vi "find device.vi"(8 "error in (no error)":errorcluster, 11 "USB-6000 in":refnum<class "USB-6000.lvclass">) -> (0 "error out":errorcluster, 3 "USB-6000 out":refnum<class "USB-6000.lvclass">)   [LabVIEW 2025, in "USB IO.lvlib" / "USB-6000.lvclass"]
uses:
  USB-6000.lvclass
  USB-6000.lvclass/USB-6000.ctl
  USB IO.lvclass
  <resource>/objmgr/daqmx.rc
panel:
  out "DO.Lines":tag[](array[tag])
  out "AI.PhysicalChans":tag[](array[tag])
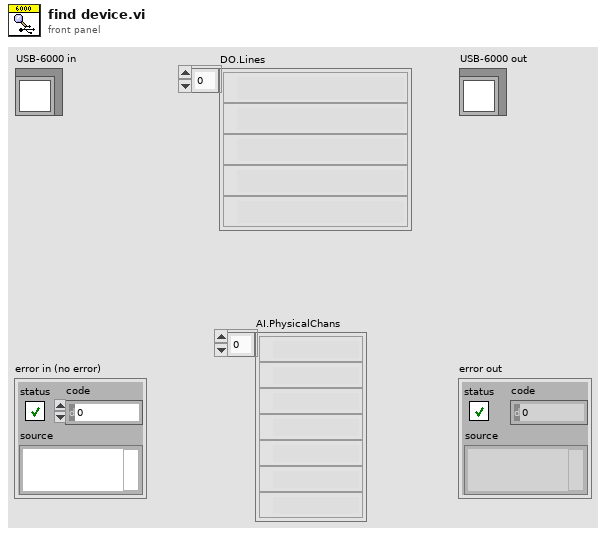
[diagram p1: front panel]
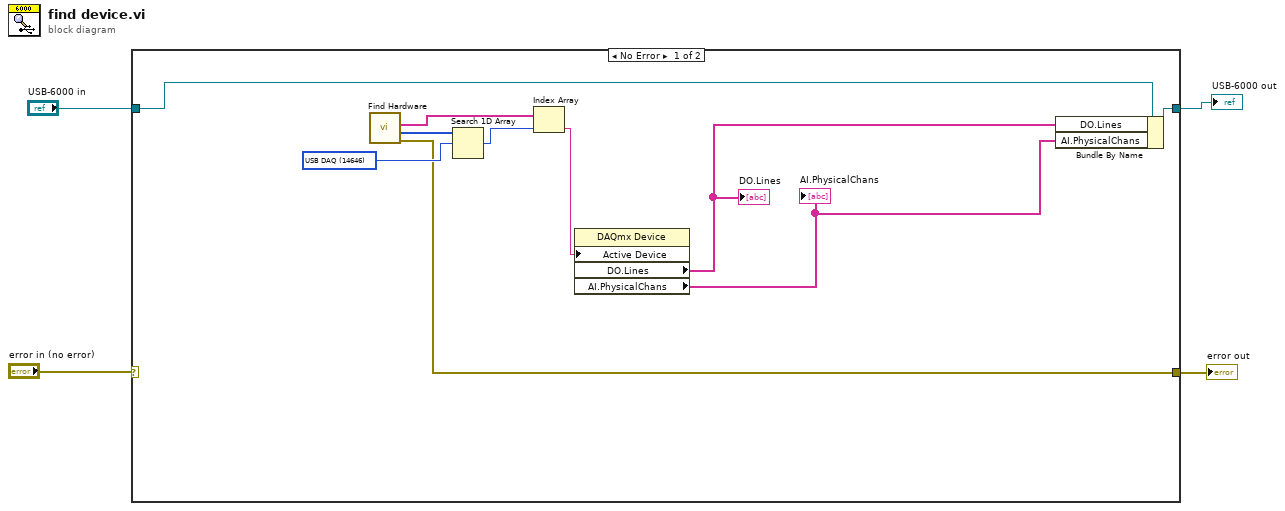
[diagram p0: block diagram]
diagram:
  n1 = case shown="No Error" "error in (no error)" {
    selector: "error in (no error)" -> [_ w16]
    tunnel: [w8 w16] -> w3
    tunnel: [w10 w15] -> w4
    tunnel: "USB-6000 in" -> [w9 w15]
    frame No Error {
      w13 = 14646 items=["M Series DAQ"=14643, "X Series DAQ"=15858, "E Series DAQ"=14642, "S Series DAQ"=14644, "B Series DAQ"=14662, "SC Series DAQ"=14645, "USB DAQ"=14646, "AO Series"=14647, "Digital I/O"=14648, "TIO Series"=14661, "Dynamic Signal Acquisition"=14649, "Switches"=14650, "CompactDAQ Chassis"=14658, "CompactRIO Chassis"=16144, "C Series Module"=14659, "SCXI Module"=14660, "SCC Connector Block"=14704, "SCC Module"=14705, "NI ELVIS"=14755, "Network DAQ"=14829, "SC Express"=15886, "FieldDAQ"=16151, "TestScale Chassis"=16180, "TestScale Module"=16181, "mioDAQ"=16182, "Unknown"=12588] ("ProductCategory")
      n2 = call "Find Hardware.vi"() -> ("error out"=w8:errorcluster, "Product Category"=w14:i32[], "DevNames"=w12:tag[])  [unwired: 8 in, 1 out]
      n3 = Search 1D Array(1D array=w14, element=w13) -> (index of element=w11:i32)  [unwired: 1 in]
      n4 = Index Array(array=w12, index=w11) -> (element=w7:tag)
      n5 = property class="DAQmx Device"("Active Device"=w7) -> ("DO.Lines"=w6:tag[], "AI.PhysicalChans"=w5:tag[])  [unwired: 2 in, 2 out]
      "DO.Lines" <- w6
      "AI.PhysicalChans" <- w5
      n6 = Bundle By Name(cluster=w9, "DO.Lines"=w6, "AI.PhysicalChans"=w5) -> (w10:refnum<class "USB-6000.lvclass">)
    }
    frame Error {
    }
  }
  "error out" <- w3
  "USB-6000 out" <- w4
